vi "NumLimitResetter.vi"(6 "LowerLimit":i32, 7 "UpperLimit":i32=22, 11 "Num In":i32) -> (3 "Num Out":i32)   [LabVIEW 2018, in "SnakeBodyCell.lvclass"]
uses:
  SnakeBodyCell.lvclass
panel:
  # "Connector Pane"
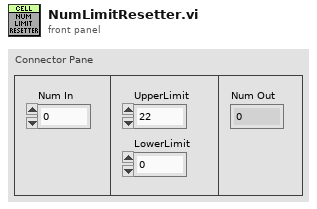
[diagram p1: front panel]
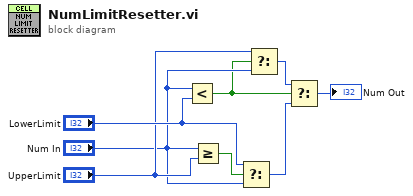
[diagram p0: block diagram]
diagram:
  n1 = Less?(x="Num In", y="LowerLimit") -> (x < y?=w4:bool)
  n2 = Greater Or Equal?(x="Num In", y="UpperLimit") -> (x >= y?=w5:bool)
  n3 = Select(t="LowerLimit", s=w5, f="Num In") -> (s? t:f=w2:i32)
  n4 = Select(t="UpperLimit", s=w4, f="Num In") -> (s? t:f=w3:i32)
  n5 = Select(t=w3, s=w4, f=w2) -> (s? t:f=→"Num Out":i32)
